vi "Reset.vi"(8 "Fehler (Eingang, kein Fehler)":errorcluster caption="Error_In", 11 "Referenz_In":refnum<visa-resource-name>) -> (0 "Fehler (Ausgang)":errorcluster caption="Error_Out", 1 "communication_data":T1, 3 "Referenz_Out":refnum<visa-resource-name>)   [LabVIEW 2018, in "OXYGEN.lvlib"]
doc: "Initializes the device to default settings."
uses:
  OXYGEN.lvlib
  TypeDefs/Cluster_RawCommData.ctl
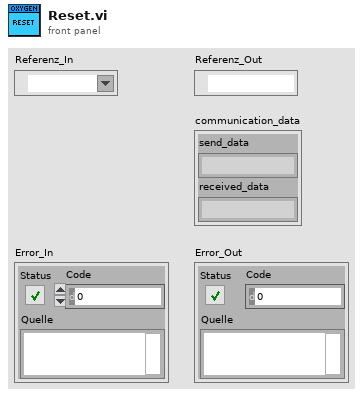
[diagram p1: front panel]
types:
  T1 = typedef "OXYGEN.lvlib/Cluster_RawCommData.ctl" = cluster{"send_data":string, "received_data":string}
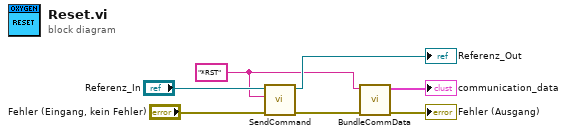
[diagram p0: block diagram]
diagram:
  w4 = "*RST" ("Schreibpuffer")
  n1 = call "SendCommand.vi"("error in (no error)"="Fehler (Eingang, kein Fehler)", "String to Send"=w4, "OXY_SCPI Reseource In"="Referenz_In") -> ("error out"=w1:errorcluster, "OXY_SCPI Reseource Out"=→"Referenz_Out":refnum<visa-resource-name>)  [unwired: 7 in]
  n2 = call "BundleCommData.vi"("error in (no error)"=w1, "send_data"=w4) -> ("error out"=→"Fehler (Ausgang)":errorcluster, "communication_data"=→"communication_data":T1)  [unwired: 8 in]
